vi "UART Set Baud Rate.vi"(8 "Error In":errorcluster, 9 "Baud Rate (9600)":u32=9600, 10 "UART Channel":u8, 11 "LINX Device Config":T1) -> (0 "Error Out":errorcluster, 3 "LINX Device Config":T1)   [LabVIEW 2011, in "LMH-LINX.lvlib" / "Device.lvlib"]
doc: "Set the buad rate of the specified UART channel."
uses:
  Device.lvlib
  Type Defs/LINX Device Config.ctl
  Type Defs/Interface.ctl
  Type Defs/TCP Config.ctl
  Type Defs/Channels.ctl
  Type Defs/Error Type.ctl
  LMH-LINX.lvlib
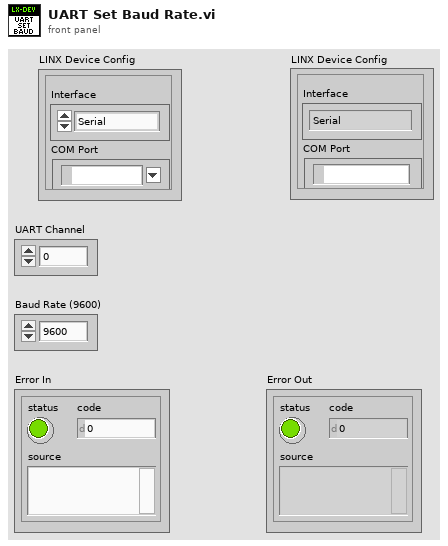
[diagram p1: front panel]
types:
  T1 = typedef "LMH-LINX.lvlib/Device.lvlib/LINX Device Config.ctl" = cluster{"Interface":T2, "COM Port":refnum<visa-resource-name>, "TCP Configuration":T3, "Device Family":u8, "Device ID":u8, "Device Name":string, "TCP Ref":refnum<k5>, "Channels":T4}
  T2 = typedef "LMH-LINX.lvlib/Interface.ctl" = enum16{"Serial", "TCP"}
  T3 = typedef "LMH-LINX.lvlib/Device.lvlib/TCP Config.ctl" = cluster{"IP Address":string, "Port":u16}
  T4 = typedef "LMH-LINX.lvlib/Channels.ctl" = cluster{"DI":u8[], "DO":u8[], "AI":u8[], "AO":u8[], "PWM":u8[], "QE":u8[], "UART":u8[], "I2C 2":u8[], "SPI":u8[], "CAN":u8[], "Servo":u8[], "AI Ref (V)":dbl, "AO Ref (V)":dbl, "AO Resolution (Bits)":u8}
  T5 = typedef "LMH-LINX.lvlib/Error Type.ctl" = enum16{"Unknown", "Timeout", "Corrupt Return Packet", "Unable To Connect", "Command Not Supported", "Channel DNE", "Invalid COM Config", "Firmware Version Mismatch", "myRIO Support", "CMD Specific Error"}
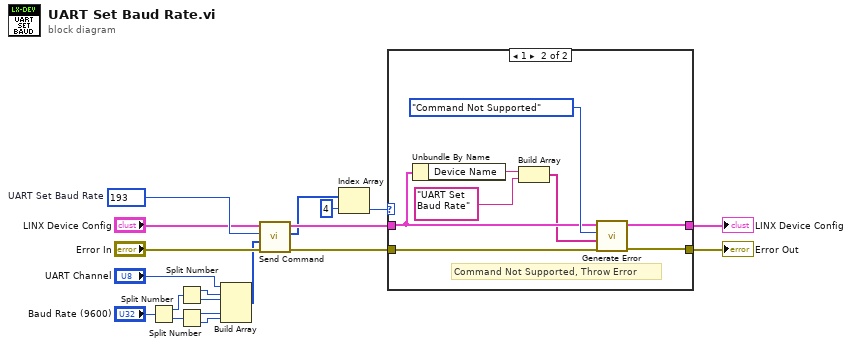
[diagram p0: block diagram]
diagram:
  w18 = u16 193  # UART Set Baud Rate
  n1 = Split Number(x="Baud Rate (9600)") -> (hi(x)=w6:u16, lo(x)=w5:u16)
  n2 = Split Number(x=w6) -> (hi(x)=w4:u8, lo(x)=w3:u8)
  n3 = Split Number(x=w5) -> (hi(x)=w2:u8, lo(x)=w1:u8)
  n4 = Build Array("UART Channel", w4, w3, w2, w1) -> (w8:u8[])
  n5 = call "Send Command.vi"("Error In"="Error In", "ARGS"=w8, "CMD"=w18, "LINX Device Config"="LINX Device Config") -> ("Error Out"=w11:errorcluster, "Response"=w10:u8[], "LINX Device Config"=w13:T1)  [unwired: 4 in, 1 out]
  n6 = Index Array(array=w10, index=4) -> (element=w15:u8)
  n7 = case shown="1" w15 {
    tunnel: [w21 w27] -> w14
    tunnel: w13 -> [w21 w23]
    tunnel: [w20 w28] -> w12
    tunnel: w11 -> [w20 w29]
    frame 0, Default {
      # "Status OK, Process Data"
    }
    frame 1 {
      # "Command Not Supported, Throw Error"
      n8 = Unbundle By Name(w23) -> ("Device Name"=w25:string)
      n9 = Build Array(w25, "UART Set Baud Rate") -> (w22:string[])
      n10 = call "Generate Error.vi"("Error In"=w29, "Arguments"=w22, "Error Type"=Error_Type."Command Not Supported", "LINX Device Config"=w23) -> ("Error Out"=w28:errorcluster, "LINX Device Config"=w27:T1)  [unwired: 6 in]
    }
  }
  "Error Out" <- w12
  "LINX Device Config" <- w14
